vi "Tahoma.vi"() -> ()   [LabVIEW 2023]
panel:
  in  "Horizontal Slide Switch":bool
  in  "Radio Buttons":enum32{"Item 0", "Item 1"}(radio)
  in  "Checkbox":bool
  in  "Knob":dbl(knob) scale=0.0..10.0
  in  "Horizontal Pointer Slide":dbl(slide) scale=0.0..10.0
  in  "Numeric":dbl
  in  "Tab Control":enum32{"Page 1", "Page 2"}(tab)
  in  "String":string="Lorem ipsum dolor sit amet, consectetur adipiscing elit, sed do eiusmod tempor incididunt ut labore et dolore magna aliqua. Ut enim ad minim veniam, quis nostrud exercitation ullamco laboris nisi ut aliquip ex ea commodo consequat. Duis aute irure dolor in reprehenderit in voluptate velit esse cillum dolore eu fugiat nulla pariatur. Excepteur sint occaecat cupidatat non proident, sunt in culpa qui officia deserunt mollit anim id est laborum."
  # "This is Screenshot"
  # "LabVIEW 2023"
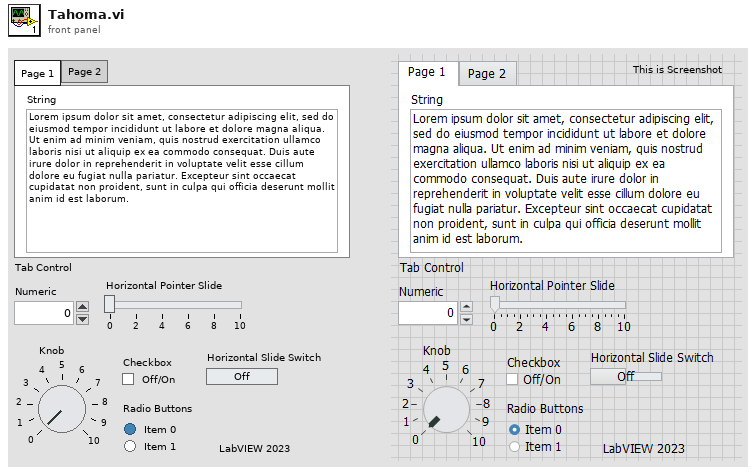
[diagram p1: front panel]
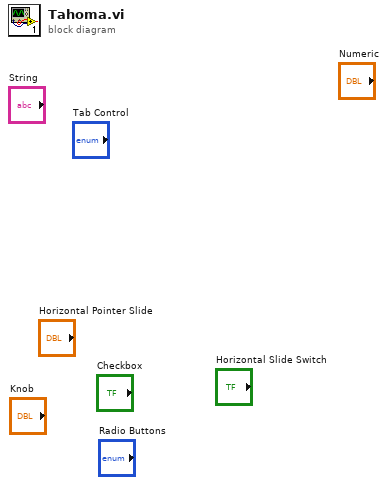
[diagram p0: block diagram]
diagram:
